vi "START VI.vi"() -> ()   [LabVIEW 2020, in "allgemeine Sub-VIs.lvlib"]
uses:
  allgemeine Sub-VIs.lvlib
  IAG-Logo-Auto B02.ctl
panel:
  in  "IAG":T1
  out "String 2":string
  out "Schieberegler":sgl(slide) scale=0.0..100.0
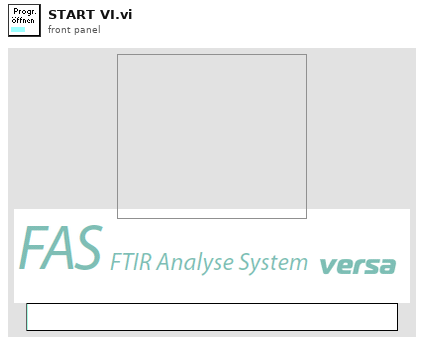
[diagram p1: front panel]
types:
  T1 = typedef "IAG-Logo-Auto B02.ctl" = bool
  T2 = enum32{"Invalid", "Standard", "Closed", "Hidden", "Minimized", "Maximized"}
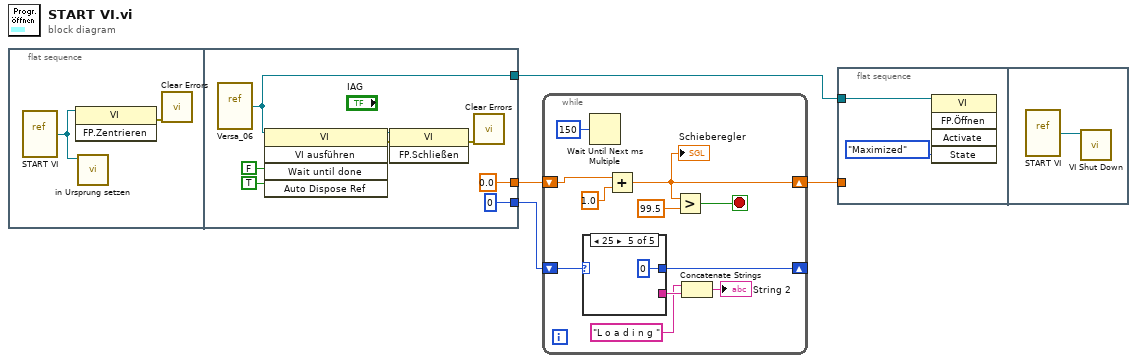
[diagram p0: block diagram]
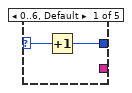
[diagram p2: hidden frame]
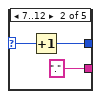
[diagram p3: hidden frame]
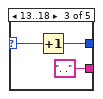
[diagram p4: hidden frame]
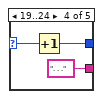
[diagram p5: hidden frame]
diagram:
  n1 = flat-sequence {
    tunnel: [sgl 0.0 ("Schieberegler")] -> w4
    tunnel: [w8] -> w3
    tunnel: [u8 0] -> w1
    frame #0 {
      n2 = vi-ref "START VI.vi"() -> (w6:refnum<vi>)
      n3 = invoke class="VI" method="FP.Zentrieren"(reference=w6) -> (error out=w5:errorcluster)  [unwired: 2 in, 2 out]
      n4 = call "in Ursprung setzen.vi"("VI Referenz"=w6) -> ()  [unwired: 11 in]
      n5 = call <vilib>:"Clear Errors.vi"("error in (no error)"=w5) -> ()  [unwired: 5 in, 2 out]
    }
    frame #1 {
      n6 = vi-ref "Versa_06.vi"() -> (w8:refnum<vi>)
      n7 = invoke class="VI" method="VI ausführen"(reference=w8, "Wait until done"=FALSE ("Warten bis beendet"), "Auto Dispose Ref"=TRUE ("Referenz automatisch schließen")) -> (reference out=w11:refnum<vi>, error out=w12:errorcluster)  [unwired: 2 in, 3 out]
      n8 = invoke class="VI" method="FP.Schließen"(reference=w11, error in=w12) -> (error out=w10:errorcluster)  [unwired: 1 in, 2 out]
      n9 = call <vilib>:"Clear Errors.vi"("error in (no error)"=w10) -> ()  [unwired: 5 in, 2 out]
    }
  }
  n10 = while {
    shift-right: [w19] -> w2
    shift-left: w4 -> [w17]
    shift-right: [w22] -> _
    shift-left: w1 -> [w23]
    stop <- w18 stop-if-true
    n11 = case shown="25" w23 {
      selector: w23 -> [w27 w30 w32 w36 _]
      tunnel: [w26 w29 w33 w35 u8 0] -> w22
      tunnel: [_ "." ". ." ". . ." _] -> w21
      frame 0..6, Default {
        n12 = Increment(x=w27) -> (x+1=w26:u8)
      }
      frame 7..12 {
        n13 = Increment(x=w30) -> (x+1=w29:u8)
      }
      frame 13..18 {
        n14 = Increment(x=w32) -> (x+1=w33:u8)
      }
      frame 19..24 {
        n15 = Increment(x=w36) -> (x+1=w35:u8)
      }
      frame 25 {
      }
    }
    n16 = Wait Until Next ms Multiple(millisecond multiple=u32 150 ("Vielfache von ms")) -> ()  [unwired: 1 out]
    n17 = Add(x=w17, y=sgl 1.0) -> (x+y=w19:sgl)
    "Schieberegler" <- w19
    n18 = Greater?(x=w19, y=sgl 99.5) -> (0:w18:bool)
    n19 = Concatenate Strings("L o a d i n g " ("String"), w21) -> (→"String 2":string)
  }
  n20 = flat-sequence {
    tunnel: w3 -> [w38]
    tunnel: w2 -> [_]
    frame #0 {
      n21 = invoke class="VI" method="FP.Öffnen"(reference=w38, "State"=T2."Maximized" ("Zustand")) -> ()  [unwired: 3 in, 5 out]
    }
    frame #1 {
      n22 = vi-ref "START VI.vi"() -> (w40:refnum<vi>)
      n23 = call "VI Shut Down.vi"("VI Referenz"=w40) -> ()  [unwired: 11 in]
    }
  }
